vi "waveform.vi"() -> ()   [LabVIEW 2023]
uses:
  <vilib>/express/express analysis/Spectral/Block/exnSpectralBlock spectral measurements RMS poly.vi
  <vilib>/express/express analysis/Spectral/XNode/ExpressSpectralMeasurementsBlockNode.xnode
  <vilib>/express/express analysis/Spectral/Block/exnSpectralBlock spectral measurements RMS DDT.vi
panel:
  in  "Boolean":bool
  in  "Ring":u16(ring) items=["Sine", "Triangle", "Square", "Sawtooth"]
  in  "Play Waveform":bool
  in  "LP Filter":dbl(slide)=1000.0 caption="Lower Cut-Off" scale=0.0..1000.0
  in  "Frequency":dbl(slide)=440.0 scale=0.0..1000.0
  out "Waveform Graph":dynamicdata(graph)
  out "Graph":dynamicdata(graph) caption="Square"
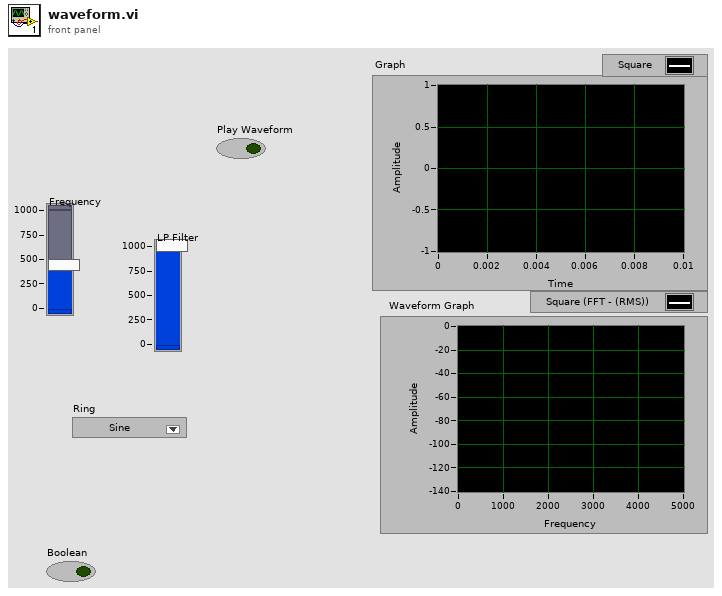
[diagram p1: front panel]
types:
  T1 = cluster{"averaging mode":u16, "weighting mode":u16, "number of averages":u32}
  T2 = cluster{"dB On (F)":bool, "unwrap phase (F)":bool, "convert to degree (F)":bool}
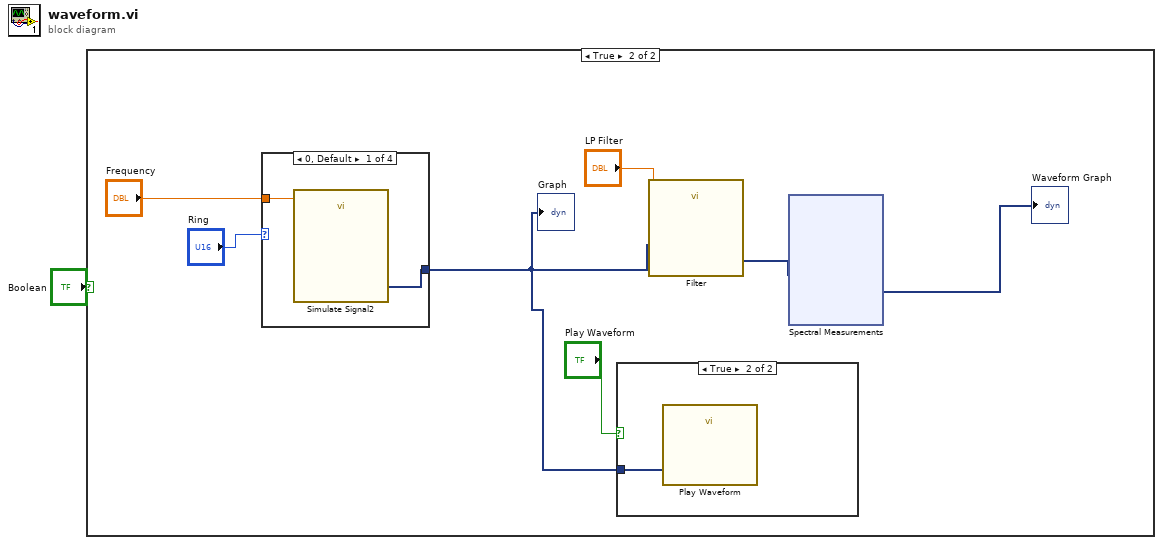
[diagram p0: block diagram]
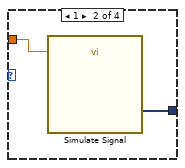
[diagram p3: hidden frame]
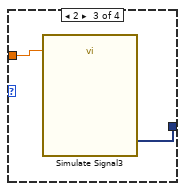
[diagram p4: hidden frame]
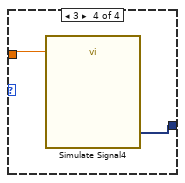
[diagram p5: hidden frame]
diagram:
  n1 = case shown="True" "Boolean" {
    frame False {
    }
    frame True {
      n2 = case shown="0, Default" "Ring" {
        tunnel: "Frequency" -> [w10 w12 w14 w16]
        tunnel: [w9 w11 w13 w15] -> w6
        frame 0, Default {
          n3 = call "Simulate Signal2"("Frequency"=w10) -> ("Sine"=w9:dynamicdata)  [unwired: 13 in, 1 out]
        }
        frame 1 {
          n4 = call "Simulate Signal"("Frequency"=w12) -> ("Triangle"=w11:dynamicdata)  [unwired: 13 in, 1 out]
        }
        frame 2 {
          n5 = call "Simulate Signal3"("Frequency"=w14) -> ("Square"=w13:dynamicdata)  [unwired: 13 in, 1 out]
        }
        frame 3 {
          n6 = call "Simulate Signal4"("Frequency"=w16) -> ("Sawtooth"=w15:dynamicdata)  [unwired: 13 in, 1 out]
        }
      }
      "Graph" <- w6
      n7 = case shown="True" "Play Waveform" {
        tunnel: w6 -> [_ w17]
        frame False {
        }
        frame True {
          n8 = call "Play Waveform"("Data"=w17) -> ()  [unwired: 18 in, 1 out]
        }
      }
      n9 = call "Filter"("Lower Cut-Off"="LP Filter", "Signal"=w6) -> ("Filtered Signal"=w4:dynamicdata)  [unwired: 8 in, 1 out]
      n10 = xnode "Spectral Measurements"("Signals"=w4) -> ("FFT - (RMS)"=→"Waveform Graph":dynamicdata)  [unwired: 1 in, 2 out]
    }
  }
